vi "Final.vi"() -> ()   [LabVIEW 2022 SP3]
uses:
  <vilib>/DAQmx/read.llb/DAQmx Read (Analog 1D DBL NChan 1Samp).vi
  <vilib>/DAQmx/write.llb/DAQmx Write (Analog DBL 1Chan 1Samp).vi
  <vilib>/DAQmx/create/channels.llb/DAQmx Create Channel (AI-Voltage-Basic).vi
  <vilib>/DAQmx/create/channels.llb/DAQmx Create Channel (AO-Voltage-Basic).vi
  <vilib>/DAQmx/miscellaneous.llb/DAQmx Fill In Error Info.vi
panel:
  in  "y":bool
  out "Temperature Indicator":dbl(knob) scale=0.0..330.0
  out "Temperature Sensor":dbl(knob) scale=0.0..3.0
  out "Boolean":bool
  in  "physical channels 2":tag
  out "Flame Sensor":dbl(knob) scale=-1.0..50.0
  out "Flame Sensor":dbl(graph)
  in  "stop":bool
  out "Gas Sensor":dbl(knob) scale=-1.0..7.0
  out "Gas Sensor":dbl(graph)
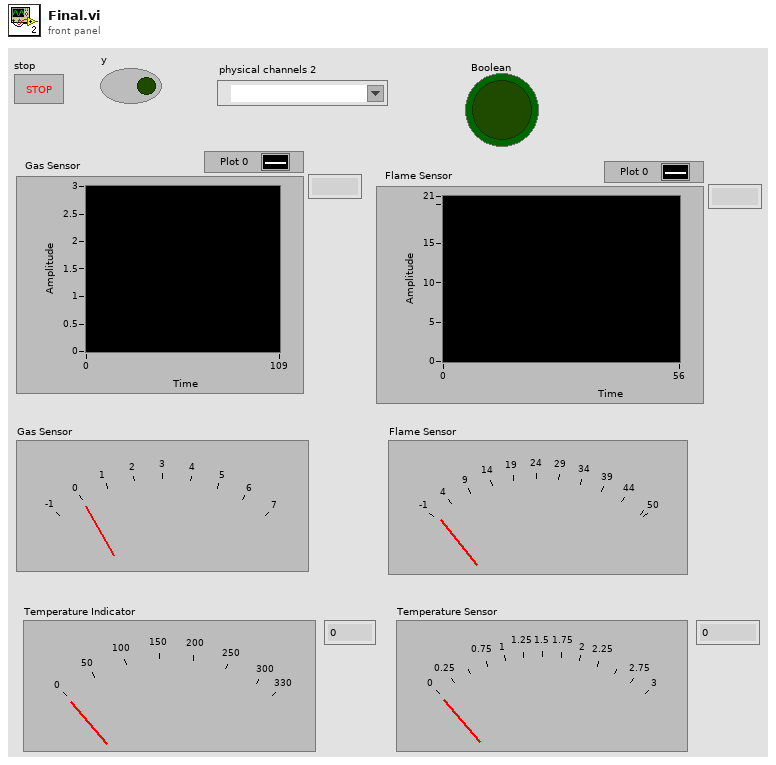
[diagram p1: front panel]
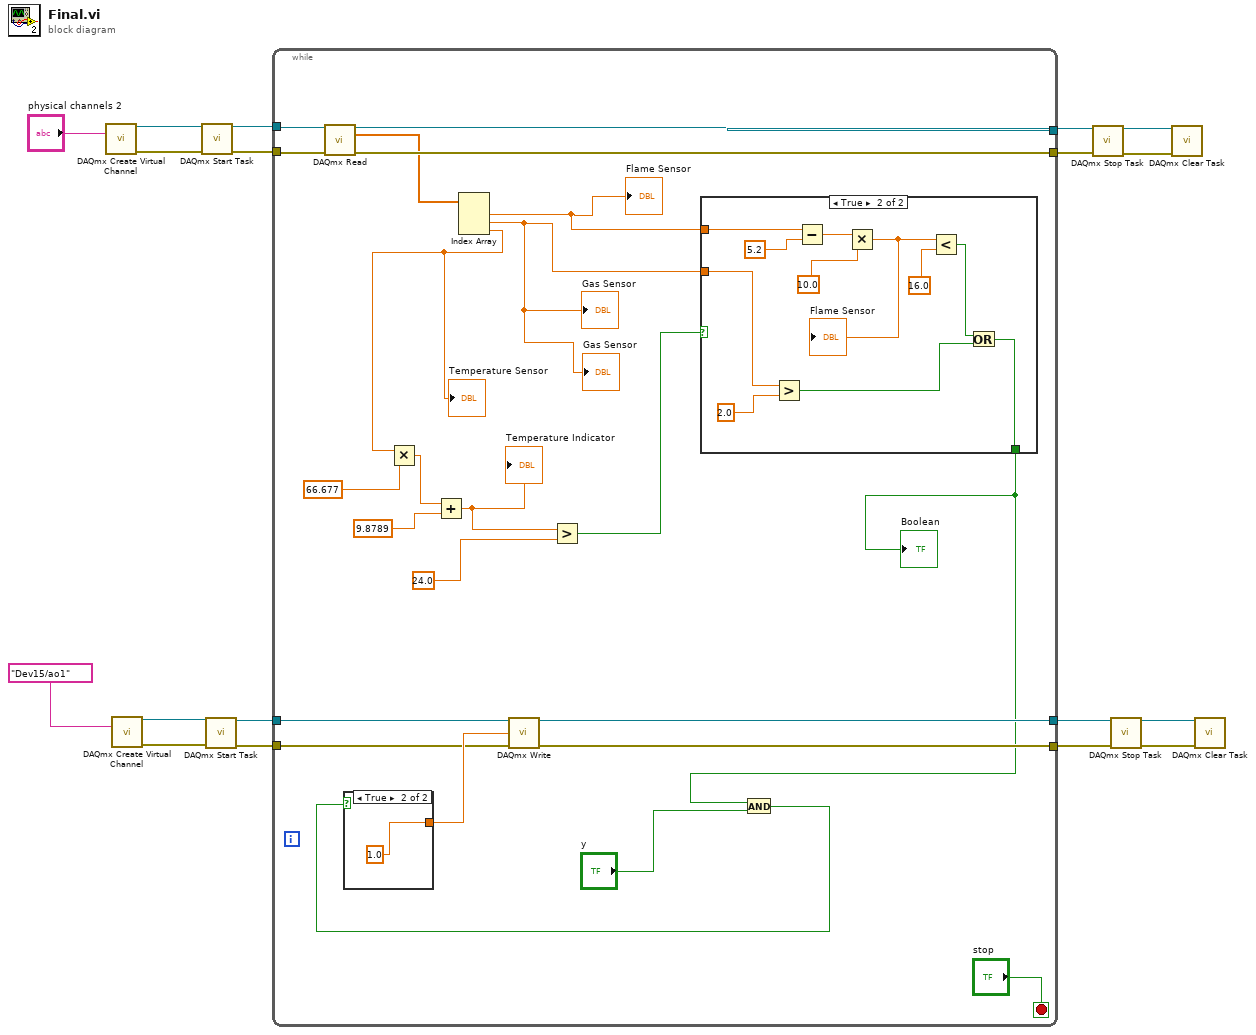
[diagram p0: block diagram]
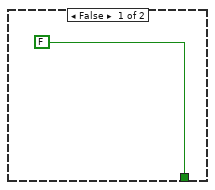
[diagram p2: hidden frame]
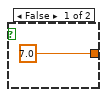
[diagram p3: hidden frame]
diagram:
  n1 = call-poly <vilib>:"DAQmx Create Virtual Channel.vi"("physical channels"="physical channels 2") -> ("task out"=w18:refnum<k21>, "error out"=w17:errorcluster)  [unwired: 13 in]
  n2 = call-poly <vilib>:"DAQmx Create Virtual Channel.vi"("physical channels"=tag "Dev15/ao1") -> ("task out"=w7:refnum<k21>, "error out"=w4:errorcluster)  [unwired: 13 in]
  n3 = call <vilib>:"DAQmx Start Task.vi"("task/channels in"=w18, "error in"=w17) -> ("task out"=w13:refnum<k21>, "error out"=w12:errorcluster)  [unwired: 12 in]
  n4 = call <vilib>:"DAQmx Start Task.vi"("task/channels in"=w7, "error in"=w4) -> ("task out"=w5:refnum<k21>, "error out"=w3:errorcluster)  [unwired: 12 in]
  n5 = while {
    tunnel: w13 -> [w38]
    tunnel: w12 -> [w37]
    tunnel: [w40] -> w11
    tunnel: [w39] -> w10
    tunnel: [w33] -> w2
    tunnel: w5 -> [w32]
    tunnel: [w20] -> w1
    tunnel: w3 -> [w21]
    stop <- "stop" stop-if-true
    n6 = call-poly <vilib>:"DAQmx Read.vi"("task/channels in"=w38, "error in"=w37) -> ("task out"=w40:refnum<k21>, "data"=w36:dbl[], "error out"=w39:errorcluster)  [unwired: 11 in]
    n7 = Index Array(array=w36) -> (element #1=w22:dbl, element #2=w28:dbl, element #3=w34:dbl)  [unwired: 3 in]
    "Gas Sensor" <- w28
    "Gas Sensor" <- w28
    "Flame Sensor" <- w22
    "Temperature Sensor" <- w34
    n8 = Multiply(x=w34, y=66.677) -> (x*y=w27:dbl)
    n9 = Add(x=w27, y=9.8789) -> (x+y=w25:dbl)
    "Temperature Indicator" <- w25
    n10 = Greater?(x=w25, y=24.0) -> (0:w29:bool)
    n11 = case shown="True" w29 {
      tunnel: w22 -> [_ w53]
      tunnel: w28 -> [_ w43]
      tunnel: [FALSE w47] -> w19
      frame False {
      }
      frame True {
        n12 = Greater?(x=w43, y=2.0) -> (0:w52:bool)
        n13 = Subtract(x=w53, y=5.2) -> (x-y=w51:dbl)
        n14 = Multiply(x=w51, y=10.0) -> (x*y=w45:dbl)
        "Flame Sensor" <- w45
        n15 = Less?(x=w45, y=16.0) -> (x < y?=w46:bool)
        n16 = Or(x=w46, y=w52) -> (x .or. y?=w47:bool)
      }
    }
    "Boolean" <- w19
    n17 = And(x=w19, y="y") -> (x .and. y?=w23:bool)
    n18 = case shown="True" w23 {
      tunnel: [7.0 1.0] -> w31
      frame False {
      }
      frame True {
      }
    }
    n19 = call-poly <vilib>:"DAQmx Write.vi"("task/channels in"=w32, "data"=w31, "error in"=w21) -> ("task out"=w33:refnum<k21>, "error out"=w20:errorcluster)  [unwired: 10 in, 1 out]
  }
  n20 = call <vilib>:"DAQmx Stop Task.vi"("task/channels in"=w11, "error in"=w10) -> ("task out"=w16:refnum<k21>, "error out"=w15:errorcluster)  [unwired: 12 in]
  n21 = call <vilib>:"DAQmx Stop Task.vi"("task/channels in"=w2, "error in"=w1) -> ("task out"=w9:refnum<k21>, "error out"=w8:errorcluster)  [unwired: 12 in]
  n22 = call <vilib>:"DAQmx Clear Task.vi"("task in"=w16, "error in"=w15) -> ()  [unwired: 13 in, 1 out]
  n23 = call <vilib>:"DAQmx Clear Task.vi"("task in"=w9, "error in"=w8) -> ()  [unwired: 13 in, 1 out]
